vi "tearDown.vi"(8 "error in (no error)":errorcluster, 11 "reference in":refnum<class "Routing and Faulting Compile Unit Tests.lvclass">) -> (0 "error out":errorcluster, 3 "reference out":refnum<class "Routing and Faulting Compile Unit Tests.lvclass">)   [LabVIEW 2017, in "Routing and Faulting Compile Unit Tests.lvclass"]
doc: "tearDown runs after the test method has completed. Use this method to clean up any operations or references that were opened by setUp or the test method. Unit tests should be independent of other unit tests so this VI should ensure that the next test can run in a 'clean' test environment."
uses:
  Routing and Faulting Compile Unit Tests.lvclass
  Routing and Faulting Compile Unit Tests.lvclass/Routing and Faulting Compile Unit Tests.ctl
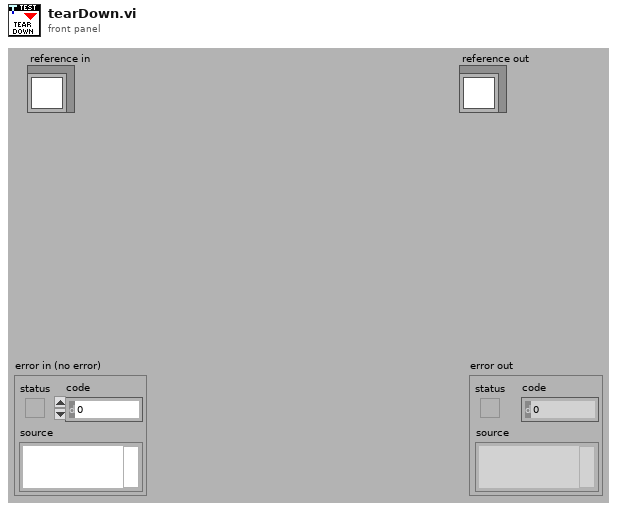
[diagram p1: front panel]
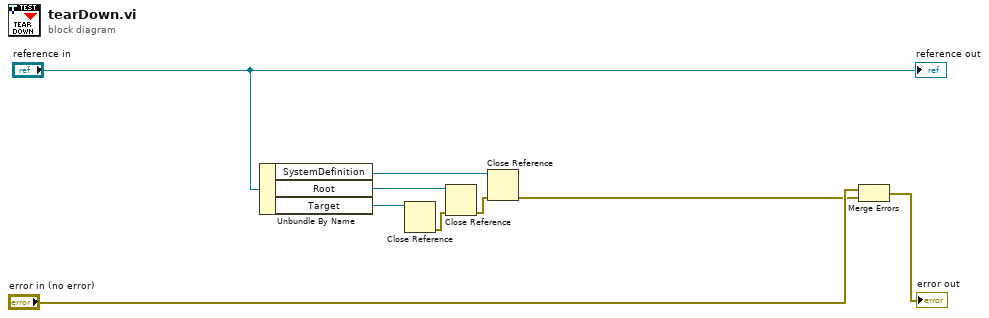
[diagram p0: block diagram]
diagram:
  n1 = Unbundle By Name("reference in") -> ("SystemDefinition"=w8:refnum<k24>, "Root"=w6:refnum<k24>, "Target"=w7:refnum<k24>)
  n2 = Close Reference(reference=w7) -> (error out=w3:errorcluster)  [unwired: 1 in]
  n3 = Close Reference(reference=w6, error in (no error)=w3) -> (error out=w5:errorcluster)
  n4 = Close Reference(reference=w8, error in (no error)=w5) -> (error out=w1:errorcluster)
  n5 = Merge Errors("error in (no error)", w1) -> (→"error out":errorcluster)
  "reference out" <- "reference in"
